vi "系统主界面 .vi"   [LabVIEW 2015]
panel:
  # "跳远系统主界系统主界面"
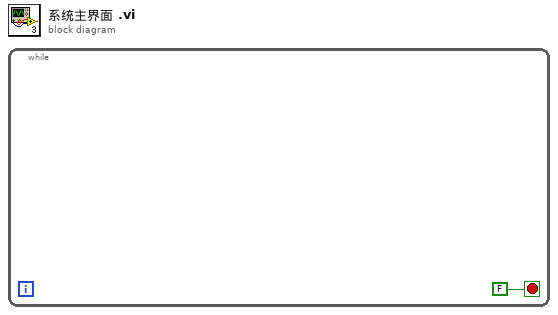
[diagram p0: block diagram]
diagram:
  n1 = while {
    stop <- FALSE stop-if-true
  }
